vi "Symphony ReadWrite test.vi"(0 "ServerIn":refnum<k13>, 1 "Lecture":bool=TRUE, 2 "Check Corresp":bool=TRUE, 3 "Read timeout ms(10000)":i32, 5 "ClientIn":refnum<k13>, 7 "URL":string="dstp://jandllab6.physique.usherbrooke.ca/", 9 "Message In":T1, 11 "ErrorIn (no error)":errorcluster caption="entrée d'erreur (pas d'erreur)", 12 "Écriture":bool=TRUE, 13 "CloseConn":bool) -> (6 "ClientOut":refnum<k13>, 10 "Data Out":T1, 15 "error out":errorcluster)   [LabVIEW 2019]
panel:
  in  "Connection":bool=TRUE
  out "chaîne de données":string
  out "données 2":variant
  out "données":cluster{string, i32}
  out "timed out":bool
  in  "stop":bool
  out "Timeout":bool
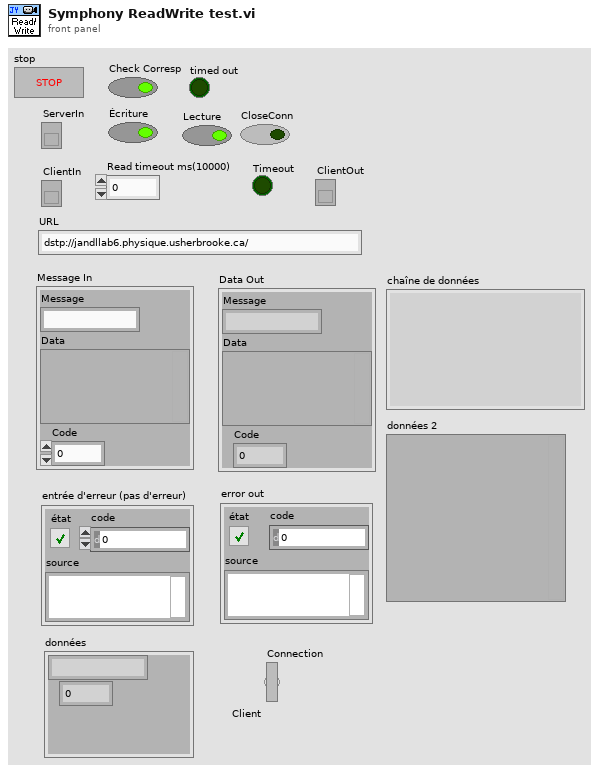
[diagram p1: front panel]
types:
  T1 = cluster{"Message":string, "Data":variant, "Code":i32}
  T2 = enum16{"Read", "Write", "ReadWrite", "BufferedRead", "BufferedReadWrite"}
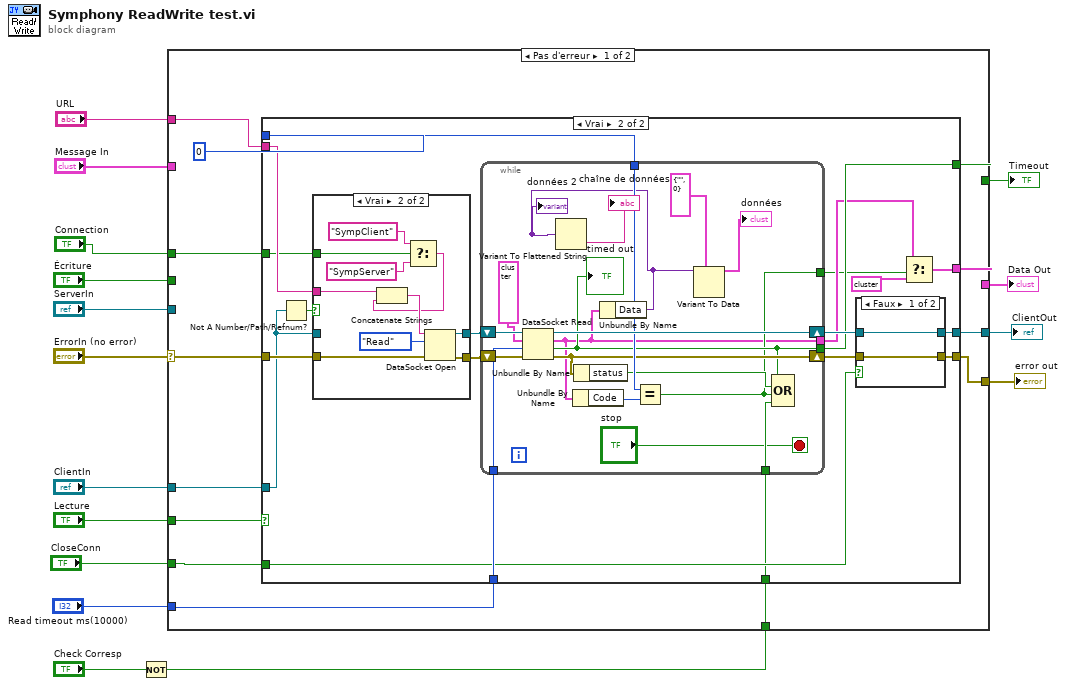
[diagram p0: block diagram]
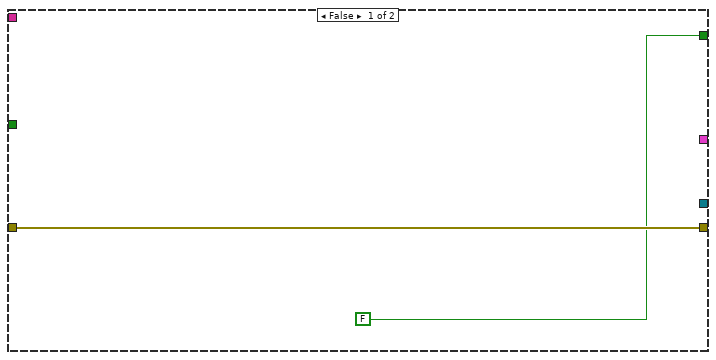
[diagram p2: hidden frame]
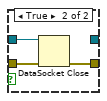
[diagram p4: hidden frame]
diagram:
  n1 = Not(x="Check Corresp") -> (.not. x?=w2:bool)
  n2 = case shown="Pas d'erreur" "ErrorIn (no error)" {
    selector: "ErrorIn (no error)" -> [w19 w87]
    tunnel: "URL" -> [w28 _]
    tunnel: "Lecture" -> [w29 _]
    tunnel: "ServerIn" -> [_ _]
    tunnel: "CloseConn" -> [w27 _]
    tunnel: "Message In" -> [_ _]
    tunnel: "ClientIn" -> [w26 _]
    tunnel: [w25 _] -> w9
    tunnel: "Read timeout ms(10000)" -> [w24 _]
    tunnel: [w23 _] -> w7
    tunnel: [w22 w87] -> w6
    tunnel: "Écriture" -> [_ _]
    tunnel: [w21 _] -> w4
    tunnel: w2 -> [w20 _]
    tunnel: "Connection" -> [w17 _]
    frame No Error {
      n3 = case shown="Vrai" w29 {
        tunnel: w19 -> [w31 w51]
        tunnel: w28 -> [_ w49]
        tunnel: [w31 w46] -> w22
        tunnel: w27 -> [_ w42]
        tunnel: w26 -> [_ w44]
        tunnel: [_ w36] -> w25
        tunnel: w24 -> [_ w43]
        tunnel: [_ w40] -> w23
        tunnel: [FALSE ("timed out") w39] -> w21
        tunnel: u32 0 ("millisecond timer value") -> [_ w38]
        tunnel: w20 -> [_ w37]
        tunnel: w17 -> [_ w32]
        frame False {
        }
        frame True {
          n4 = Not A Number/Path/Refnum?(number/path/refnum=w44) -> (NaN/Path/Refnum?=w45:bool)
          n5 = case shown="Vrai" w45 {
            tunnel: w51 -> [w70 w81]
            tunnel: [w70 w80] -> w50
            tunnel: w49 -> [_ w79]
            tunnel: [w71 w76] -> w48
            tunnel: w44 -> [w71 _]
            tunnel: w32 -> [_ w72]
            frame False {
            }
            frame True {
              n6 = Select(t="SympClient", s=w72, f="SympServer") -> (s? t:f=w73:string)
              n7 = Concatenate Strings(w79, w73) -> (w78:string)
              n8 = DataSocket Open(8:w81, 10:T2."Read" ("mode"), 11:w78) -> (0:w80:errorcluster, 3:w76:refnum<k13>)  [unwired: 1 in]
            }
          }
          n9 = while {
            tunnel: [w53] -> w35
            tunnel: w43 -> [w67]
            tunnel: [w60] -> w39
            shift-right: [w62] -> w47
            shift-left: w50 -> [w69]
            shift-right: [w66] -> w41
            shift-left: w48 -> [w68]
            tunnel: w38 -> [w64]
            tunnel: w37 -> [w63]
            tunnel: [w59] -> w34
            stop <- "stop" stop-if-true
            n10 = DataSocket Read(8:w69, 9:w67, 10:T1 {"Message"="", "Data"=variant, "Code"=0}, 11:w68) -> (0:w62:errorcluster, 1:w60:bool, 2:w53:T1, 3:w66:refnum<k13>)  [unwired: 1 in, 3 out]
            "timed out" <- w60
            n11 = Unbundle By Name(w53) -> ("Code"=w65:i32)
            n12 = Unbundle By Name(w62) -> ("status"=w61:bool)
            n13 = Unbundle By Name(w53) -> ("Data"=w52:variant)
            "données 2" <- w52
            n14 = Variant To Flattened String(Variant=w52) -> (data string=→"chaîne de données":string)  [unwired: 1 out]
            n15 = Equal?(x=w64, y=w65) -> (x = y?=w59:bool)
            n16 = Variant To Data(type=cluster{string, i32} {"", 0}, Variant=w52) -> (data=→"données":cluster{string, i32})  [unwired: 1 in, 1 out]
            n17 = Compound Arithmetic op=OR ("Opérateur arithmétique")(w60, w61, w59, w63) -> ()  [unwired: 1 out]
          }
          n18 = case shown="Faux" w42 {
            tunnel: w47 -> [w83 w86]
            tunnel: [w83 w85] -> w46
            tunnel: w41 -> [w82 w84]
            tunnel: [w82 _] -> w40
            frame False {
            }
            frame True {
              n19 = DataSocket Close(8:w86, 11:w84) -> (0:w85:errorcluster)  [unwired: 1 in, 1 out]
            }
          }
          n20 = Select(t=w35, s=w34, f=T1 {"Message"="CommError", "Data"=variant, "Code"=0} ("cas faux")) -> (s? t:f=w36:T1)
        }
      }
    }
    frame Error {
    }
  }
  "Data Out" <- w9
  "ClientOut" <- w7
  "error out" <- w6
  "Timeout" <- w4
